vi "Empty Hardware Configuration.vi"() -> (0 "Hardware Configuration":T1)   [LabVIEW 2021, in "Acquisition.lvlib"]
doc: "(inline VI) Return an empty Hardware Configuration value. Use in-place of a block diagram constant.\n\nA cluster that holds the all of the settings for data acquisition, including channels and timing."
uses:
  Acquisition.lvlib
  Hardware Configuration.ctl
  Channel Settings.ctl
  IO Device.ctl
  Sensor Type.ctl
  Interval Timer/Repeat Interval.ctl
  Interval Timer/Interval Length.ctl
  Interval Timer/Interval Token.ctl
  IO API.ctl
  Interval Timer/Interval Timer.lvlib
  IO Context.ctl
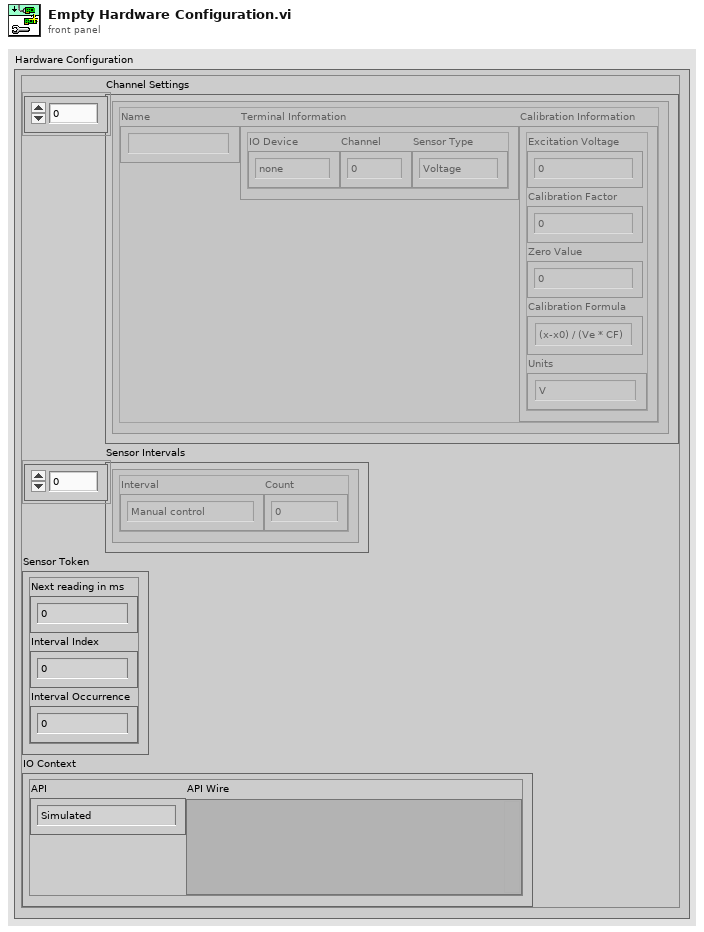
[diagram p1: front panel]
types:
  T1 = typedef "Acquisition.lvlib/Hardware Configuration.ctl" = cluster{"Channel Settings":T2[], "Sensor Intervals":T5[], "Sensor Token":T7, "IO Context":T8}
  T2 = typedef "Acquisition.lvlib/Channel Settings.ctl" = cluster{"Name":string, "Terminal Information":cluster{"IO Device":T3, "Channel":i32, "Sensor Type":T4}, "Calibration Information":cluster{"Excitation Voltage":dbl, "Calibration Factor":dbl, "Zero Value":dbl, "Calibration Formula":string, "Units":string}}
  T3 = typedef "Acquisition.lvlib/IO Device.ctl" = enum16{"none", "9219", "9401"}
  T4 = typedef "Acquisition.lvlib/Sensor Type.ctl" = enum16{"Voltage", "Load", "Pressure", "Encoder"}
  T5 = typedef "Interval Timer.lvlib/Repeat Interval.ctl" = cluster{"Interval":T6, "Count":i32}
  T6 = typedef "Interval Timer.lvlib/Interval Length.ctl" = enum16{"Manual control", "1 second", "10 seconds", "30 seconds", "60 seconds", "600 seconds", "1200 seconds", "3600 seconds"}
  T7 = typedef "Interval Timer.lvlib/Interval Token.ctl" = cluster{"Next reading in ms":u32, "Interval Index":i32, "Interval Occurrence":i32}
  T8 = typedef "Acquisition.lvlib/IO Context.ctl" = cluster{"API":T9, "API Wire":variant}
  T9 = typedef "Acquisition.lvlib/IO API.ctl" = enum16{"Simulated", "DAQmx"}
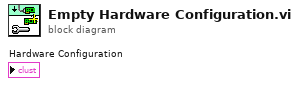
[diagram p0: block diagram]
diagram:
